vi "InitSettings.vi"(8 "error in (no error)":errorcluster, 10 "refs":T1, 11 "Config":refnum<class "Config.lvclass">) -> (0 "error out":errorcluster, 3 "Config":refnum<class "Config.lvclass">)   [LabVIEW 2014, in "Framework.lvlib" / "Config.lvclass"]
uses:
  Config.lvclass
  Typedefs/clSettingsRefs.ctl
  Config.lvclass/Config.ctl
  Accessors/Read PARTF Root Directory.vi
  Read Logging.vi
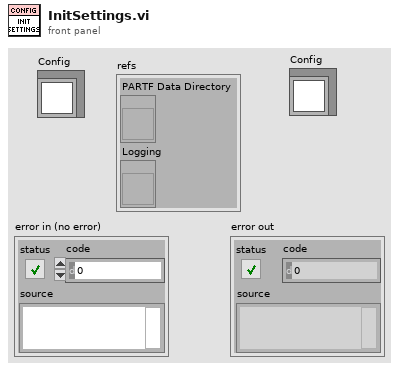
[diagram p1: front panel]
types:
  T1 = typedef "Framework.lvlib/Config.lvclass/clSettingsRefs.ctl" = cluster{"PARTF Data Directory":refnum<vi>, "Logging":refnum<vi>}
  T2 = typedef "Framework.lvlib/Config.lvclass/RootDir.ctl" = cluster{"pathRootDir":path, "btnOutPath":bool, "OutDir":string, "btnOpenOutputDir":bool, "ScriptDir":string, "btnOpenScriptDir":bool, "TestDir":string, "btnOpenTestDir":bool}
  T3 = typedef "Framework.lvlib/Config.lvclass/Logging.ctl" = cluster{"eLogLvl":T4, "Log File Path":path, "btnLogFile":bool}
  T4 = typedef "Framework.lvlib/Config.lvclass/eLogLvl.ctl" = enum16{"Normal", "Verbose", "None"}
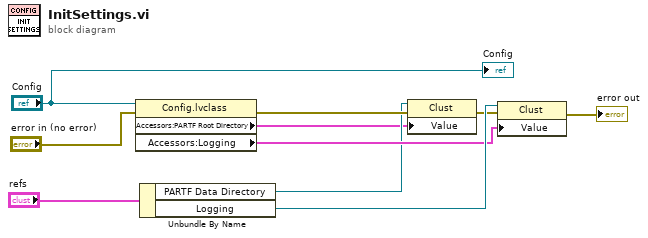
[diagram p0: block diagram]
diagram:
  n1 = property class="Config.lvclass"(reference="Config", error in="error in (no error)") -> (error out=w8:errorcluster, "Accessors:PARTF Root Directory"=w1:T2, "Accessors:Logging"=w3:T3)  [unwired: 1 out]
  n2 = Unbundle By Name("refs") -> ("PARTF Data Directory"=w2:refnum<vi>, "Logging"=w9:refnum<vi>)
  n3 = property class="Clust"(reference=w2, error in=w8, "Value"=w1) -> (error out=w7:errorcluster)  [unwired: 1 out]
  n4 = property class="Clust"(reference=w9, error in=w7, "Value"=w3) -> (error out=→"error out":errorcluster)  [unwired: 1 out]
  "Config" <- "Config"
